vi "Serial Number Entering.vi"(11 "Number of Units":i32) -> (3 "Serial Numbers":string[](array[string]))   [LabVIEW 2023]
panel:
  in  "Enter":bool
  in  "Serial Number":string
  out "Total Units":i32
  out "Current Unit":i32
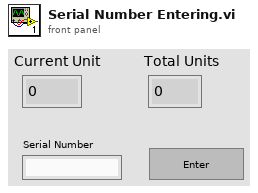
[diagram p1: front panel]
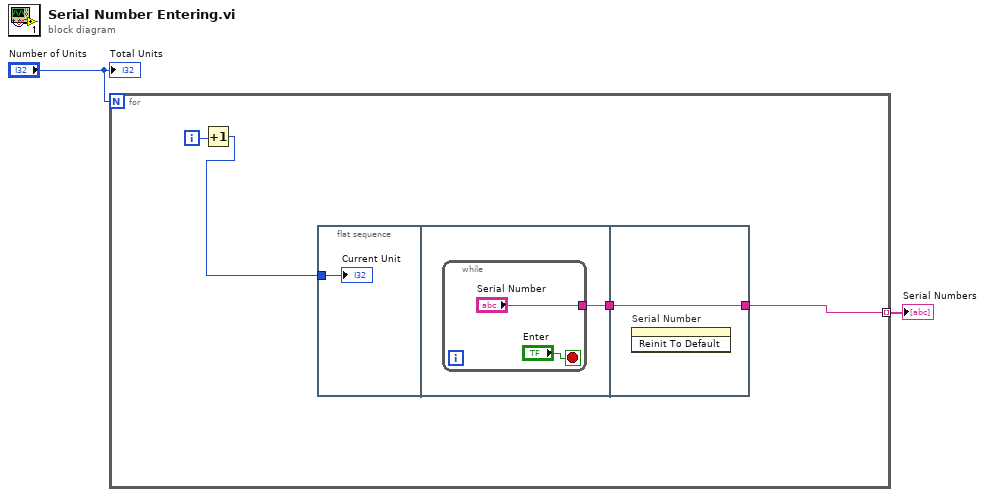
[diagram p0: block diagram]
diagram:
  n1 = for {
    N: "Number of Units" -> [_]
    tunnel: [w4] -> w1 mode=indexing
    i -> [w6]
    n2 = Increment(x=w6) -> (x+1=w5:i32)
    n3 = flat-sequence {
      tunnel: w5 -> [w7]
      tunnel: [w8] -> w3
      tunnel: [w11] -> w4
      tunnel: w3 -> [w11]
      frame #0 {
        "Current Unit" <- w7
      }
      frame #1 {
        n4 = while {
          tunnel: ["Serial Number"] -> w8
          stop <- "Enter" stop-if-true
        }
      }
      frame #2 {
        n5 = invoke on="Serial Number" class="Str" method="Reinit To Default"() -> ()  [unwired: 3 in, 3 out]
      }
    }
  }
  "Serial Numbers" <- w1
  "Total Units" <- "Number of Units"
